vi "Set Platform Plugins.vi"(8 "error in (no error)":errorcluster, 10 "Platform Plugins":refnum<class "PlatformManager.lvclass">, 11 "PlatformListPanel in":refnum<class "PlatformListPanel.lvclass">) -> (0 "error out":errorcluster, 3 "PlatformListPanel out":refnum<class "PlatformListPanel.lvclass">)   [LabVIEW 2020, in "PicoG-App.lvlib" / "PlatformListPanel.lvclass"]
uses:
  PlatformListPanel.lvclass
  PlatformListPanel.lvclass/PlatformListPanel.ctl
  Builds/picoG/ppl/PicoG-Core.lvlibp/PicoG-Processor/PicoG-Core/PlatformPluginManager/PlatformManager.lvclass
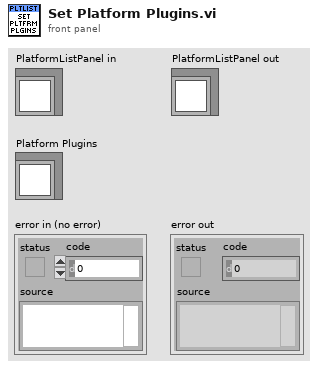
[diagram p1: front panel]
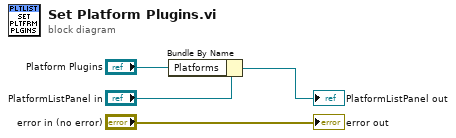
[diagram p0: block diagram]
diagram:
  n1 = Bundle By Name(cluster="PlatformListPanel in", "Platforms"="Platform Plugins") -> (→"PlatformListPanel out":refnum<class "PlatformListPanel.lvclass">)
  "error out" <- "error in (no error)"
